vi "Read station.vi"(8 "error in (no error)":errorcluster, 11 "Inovance3UTcp in":refnum<class "InovanceModbusTcp.lvclass">) -> (0 "error out":errorcluster, 2 "station":u8, 3 "Inovance3UTcp out":refnum<class "InovanceModbusTcp.lvclass">)   [LabVIEW 2020, in "HslCommunication.lvlib" / "InovanceModbusTcp.lvclass"]
uses:
  InovanceModbusTcp.lvclass
  InovanceModbusTcp.lvclass/InovanceModbusTcp.ctl
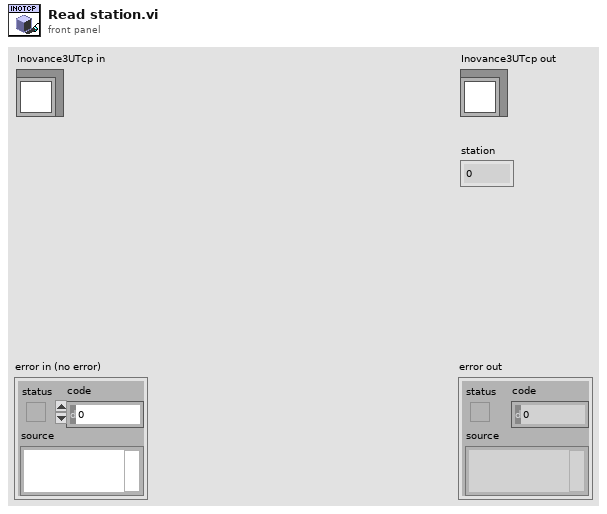
[diagram p1: front panel]
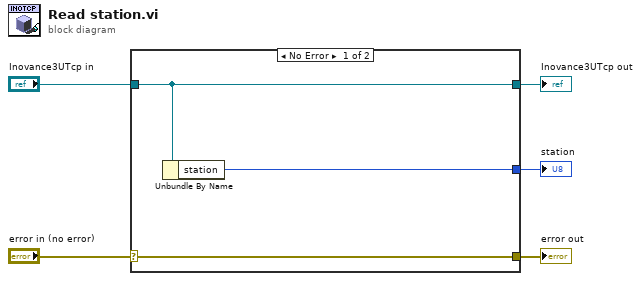
[diagram p0: block diagram]
diagram:
  n1 = case shown="No Error" "error in (no error)" {
    selector: "error in (no error)" -> [w8 w9]
    tunnel: [w8 w9] -> w4
    tunnel: [w7 w10] -> w2
    tunnel: "Inovance3UTcp in" -> [w7 w10]
    tunnel: [w6 _] -> w1
    frame No Error {
      n2 = Unbundle By Name(w7) -> ("station"=w6:u8)
    }
    frame Error {
    }
  }
  "error out" <- w4
  "Inovance3UTcp out" <- w2
  "station" <- w1
